vi "LJM_StreamBurst2D.vi"(0 "Handle In":i32, 1 "aScanList":i32[](array[numeric]), 5 "NumScans":i32, 7 "NumAddresses (-1 = Auto-Detect)":i32=-1, 9 "ScanRate":dbl format="%_2f", 11 "error in":errorcluster) -> (4 "Handle Out":i32, 6 "aData Out":dbl[][](array[numeric]), 15 "error out":errorcluster)   [LabVIEW 2020]
uses:
  Library/Frameworks/LabJackM.framework
panel:
  # "If NumAddresses = -1, then the NumAddresses control is ignored and the\nsize of aScanList is used to determine how many addresses there are."
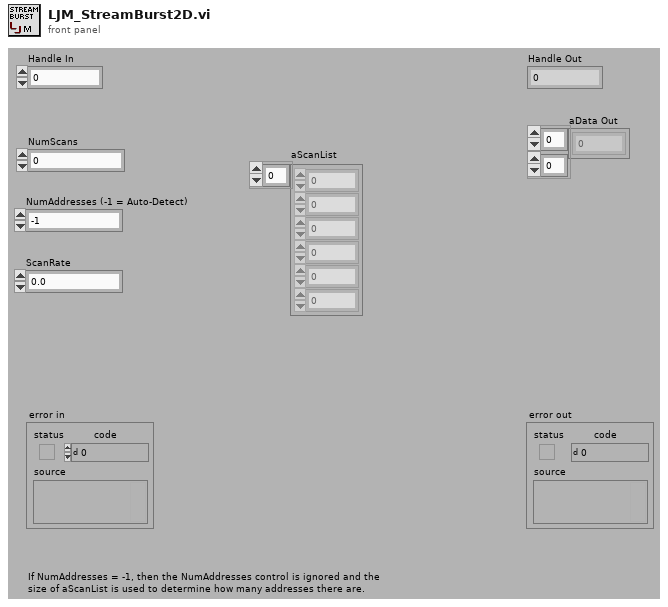
[diagram p1: front panel]
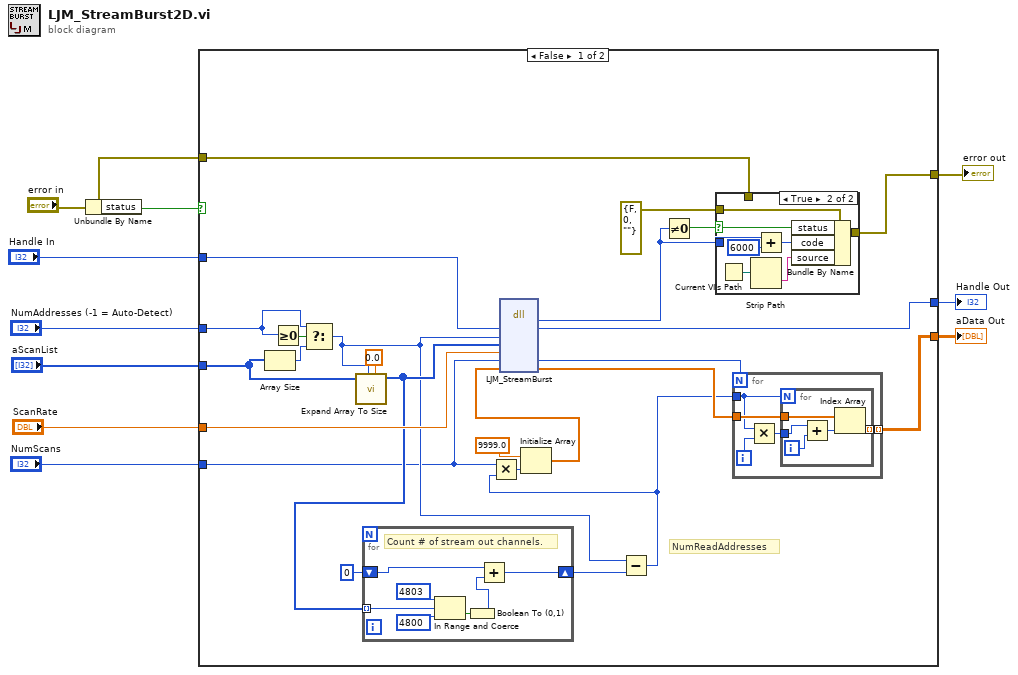
[diagram p0: block diagram]
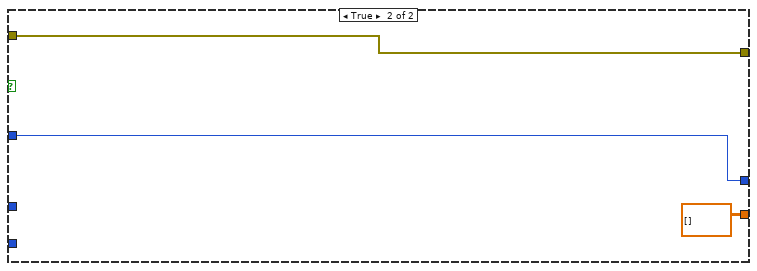
[diagram p3: hidden frame]
diagram:
  n1 = Unbundle By Name("error in") -> ("status"=w10:bool)
  n2 = case shown="False" w10 {
    tunnel: "error in" -> [w31 w64]
    tunnel: [w32 w64] -> w9
    tunnel: [w30 w63] -> w8
    tunnel: "Handle In" -> [w29 w63]
    tunnel: [w28 dbl[][] []] -> w6
    tunnel: "NumAddresses (-1 = Auto-Detect)" -> [w24 _]
    tunnel: "aScanList" -> [w23 _]
    tunnel: "ScanRate" -> [w22 _]
    tunnel: "NumScans" -> [w14 _]
    frame False {
      # "NumReadAddresses"
      n3 = Array Size(array=w23) -> (size(s)=w27:i32)
      n4 = Greater Or Equal To 0?(x=w24) -> (x >= 0?=w26:bool)
      n5 = Select(t=w24, s=w26, f=w27) -> (s? t:f=w16:i32)
      n6 = call "Expand Array To Size.vi"("Default Value"=0.0, "# Elements"=w16, "I32 Array In"=w23) -> ("I32 Array Out"=w17:i32[])  [unwired: 4 in, 4 out]
      n7 = for {
        tunnel: w17 -> [w42] mode=indexing
        shift-right: [w38] -> w15
        shift-left: i16 0 -> [w36]
        # "Count # of stream out channels."
        n8 = In Range and Coerce(upper limit=4803, x=w42, lower limit=4800) -> (In Range?=w39:bool)  [unwired: 1 out]
        n9 = Boolean To (0,1)(Boolean=w39) -> (0, 1=w37:i16)
        n10 = Add(x=w36, y=w37) -> (x+y=w38:i16)
      }
      n11 = Subtract(x=w16, y=w15) -> (x-y=w12:i32)
      n12 = Multiply(x=w14, y=w12) -> (x*y=w20:i32)
      n13 = Initialize Array(9999.0 ("element"), w20) -> (w13:dbl[])
      n14 = dll-call lib="Library/Frameworks/LabJackM.framework" fn="LJM_StreamBurst"("Handle"=w29, "NumAddresses"=w16, "aScanList"=w17, "ScanRate"=w22, "NumScans"=w14, "aData"=w13) -> ("return type"=w35:i32, "Handle"=w30:i32, "NumScans"=w11:u32, "aData"=w21:dbl[])  [unwired: 6 in, 2 out]
      n15 = Not Equal To 0?(x=w35) -> (x != 0?=w34:bool)
      n16 = case shown="True" w34 {
        selector: w34 -> [_ w60]
        tunnel: [w53 w61] -> w32
        tunnel: errorcluster {"status"=FALSE, "code"=0, "source"=""} ("error IO") -> [_ w59]
        tunnel: w35 -> [_ w55]
        tunnel: w31 -> [w53 _]
        frame False {
        }
        frame True {
          n17 = Current VI's Path() -> (path=w57:path)
          n18 = Strip Path(path=w57) -> (name=w58:string)  [unwired: 1 out]
          n19 = Add(x=w55, y=6000) -> (x+y=w56:i32)
          n20 = Bundle By Name(cluster=w59, "status"=w60, "code"=w56, "source"=w58) -> (w61:errorcluster)
        }
      }
      n21 = for {
        N: w11 -> [_]
        tunnel: w12 -> [w45]
        tunnel: w21 -> [w47]
        tunnel: [w43] -> w28 mode=indexing
        i -> [w46]
        n22 = Multiply(x=w45, y=w46) -> (x*y=w44:i32)
        n23 = for {
          N: w45 -> [_]
          tunnel: w47 -> [w52]
          tunnel: w44 -> [w49]
          tunnel: [w48] -> w43 mode=indexing
          i -> [w50]
          n24 = Add(x=w49, y=w50) -> (x+y=w51:i32)
          n25 = Index Array(array=w52, index=w51) -> (element=w48:dbl)
        }
      }
    }
    frame True {
    }
  }
  "error out" <- w9
  "Handle Out" <- w8
  "aData Out" <- w6
